vi "TurnCCW2Angle.vi"   [LabVIEW 2016, in "Project 2 LabVIEW.lvrbt"]
uses:
  Project 2 LabVIEW.lvrbt
  <vilib>/NXT/Block Support/NXT_OutputPort.ctl
  <vilib>/NXT/NXTIO Xnodes/NXTIONodeSubVIs/NXTMoveMotors.vi
  <vilib>/NXT/Dual Mode Library/Waits/Wait_Num.vi
  <vilib>/NXT/NXTIO Xnodes/NXTIONodeSubVIs/NXTStopMotors.vi
  <vilib>/NXT/Subs/LVHSConnector.ctl
  <vilib>/NXT/NXTIO Xnodes/AddressXNode/NXTIOAddress.xnode
  <vilib>/NXT/NXTIO Xnodes/NXTIOXNode/NXTIO.xnode
  <vilib>/NXT/LegoClasses/BrickReference/BrickReference.lvclass
types:
  T1 = typedef "NXT_OutputPort.ctl" = u8
  T2 = typedef "LVHSConnector.ctl" = refnum<class "BrickReference.lvclass">
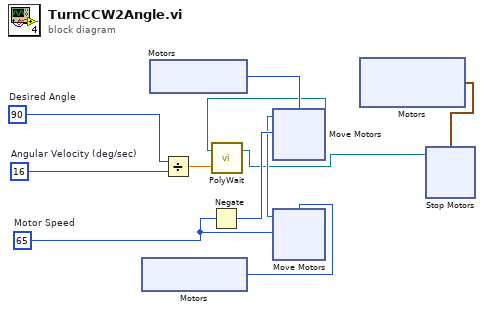
[diagram p0: block diagram]
diagram:
  w6 = 65  # Motor Speed
  w11 = 90  # Desired Angle
  w10 = 16  # Angular Velocity (deg/sec)
  n1 = xnode "Motors"() -> ("Motor"=w7:T1)
  n2 = xnode "Motors"() -> ("Motor"=w8:T1)
  n3 = Divide(x=w11, y=w10) -> (x/y=w9:dbl)
  n4 = Negate(x=w6) -> (-x=w5:i32)
  n5 = xnode "Move Motors"("Power/Speed 1"=w6, "Motors"=w7) -> ("NXT/EV3"=w3:T2)  [unwired: 1 in]
  n6 = xnode "Move Motors"("Power/Speed 1"=w5, "Motors"=w8, "NXT/EV3"=w3) -> ("NXT/EV3"=w4:T2)
  n7 = call-poly <vilib>:"PolyWait.vi"("Time (1 sec)"=w9, "NXT/EV3"=w4) -> ("NXT/EV3"=w2:T2)  [unwired: 2 in]
  n8 = xnode "Motors"() -> ("Motor"=w1:cluster{"Port":T1, "Port":T1})
  n9 = xnode "Stop Motors"("Motors"=w1, "NXT/EV3"=w2) -> ()  [unwired: 1 out]
